vi "rawcdc_protocol.vi"() -> ()   [LabVIEW 2024]
doc: "This example performs writes and reads on a serial port, as directed by the user. You can press the Write and Read buttons, and change the Read Count, while the example is running.\n\nThe parameters set for the serial port must match the parameters of the connected instrument or device. In this example, the Read Count parameter specifies the number of bytes that the serial port reads. If there were more bytes at the port than the specified number, those bytes would not be read. If there were less bytes at the port than the specified number, you would receive a timeout error.\n\nThis example expands upon the flow control options for XON and XOFF, allowing the user to choose those control characters. Also, the user can enable or disable a termination character. Some devices require a termination character in order to identify the end of command strings. Some devices send a termination character to signify the end of data to be read. This example shows how you can end the Read operation once a termination character is detected in the buffer and/or append a termination character at the end of the Write data."
uses:
  <vilib>/Instr/_visa.llb/VISA Configure Serial Port (Instr).vi
panel:
  in  "Correction":dbl(slide) scale=-10.0..10.0
  in  "index (row)":i32
  in  "Cal Array":dbl[][](array[numeric])
  out "Scaled":dbl
  out "Measured":dbl
  out "Waveform Chart":dbl[](graph)
  in  "Command List":string="stop\nencode 0\nslist 0 0\nsrate 6000\nps 2\ndec 1\ndeca 3\nnop\n\n\n"
  in  "Stop":bool
  in  "2108 CDC Virtual COM":refnum<visa-resource-name>="COM11"
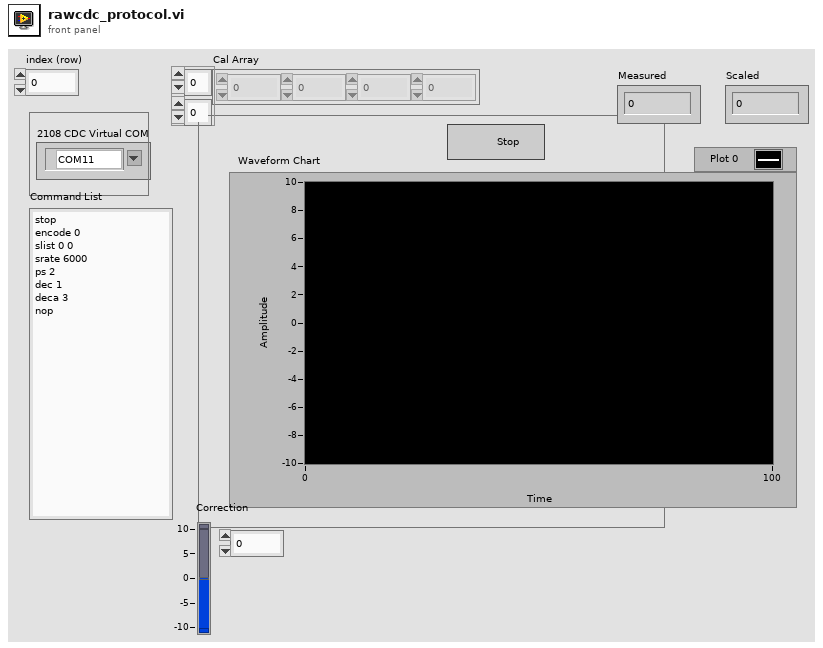
[diagram p1: front panel]
types:
  T1 = enum16{"big-endian, network order", "native, host order", "little-endian"}
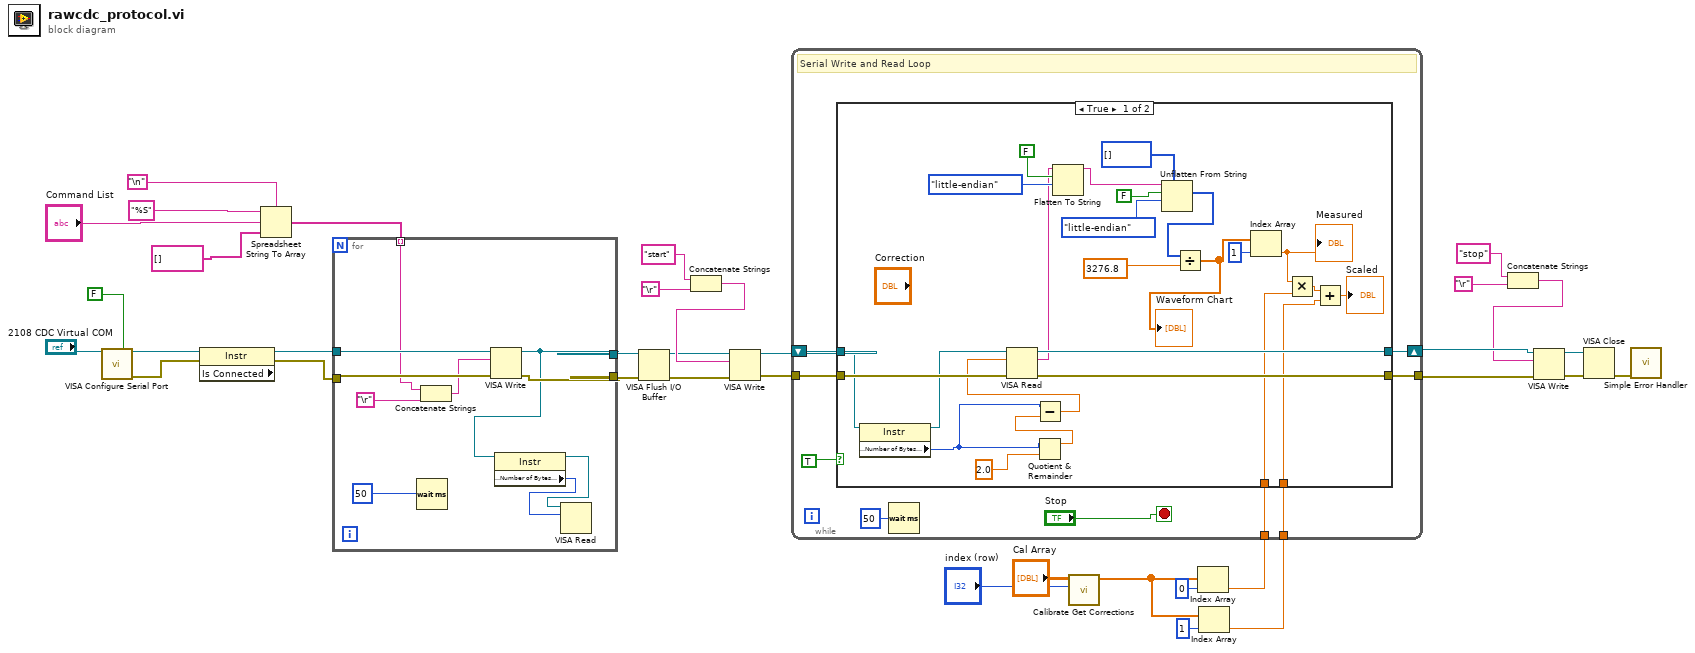
[diagram p0: block diagram]
diagram:
  n1 = call-poly "VISA Configure Serial Port"("VISA resource name"="2108 CDC Virtual COM", "Enable Termination\nChar (T)"=FALSE) -> ("VISA resource name out"=w33:refnum<visa-resource-name>, "error out"=w35:errorcluster)  [unwired: 8 in, 4 out]
  n2 = property class="Instr" props=["Is Connected"](reference=w33, error in=w35) -> (reference out=w9:refnum<visa-resource-name>, error out=w8:errorcluster)  [unwired: 1 out]
  n3 = Spreadsheet String To Array(delimiter (Tab)="\n", format string="%S", spreadsheet string="Command List", array type (2D Dbl)=string[] []) -> (array=w29:string[])
  n4 = for {
    tunnel: w29 -> [w42] mode=indexing
    tunnel: w9 -> [w45]
    tunnel: w8 -> [w44]
    tunnel: [w38] -> w13
    tunnel: [w39] -> w11
    n5 = Wait (ms)(milliseconds to wait=u32 50) -> ()  [unwired: 1 out]
    n6 = Concatenate Strings(w42, "\r") -> (w40:string)
    n7 = VISA Write(VISA resource name=w45, write buffer=w40, error in (no error)=w44) -> (VISA resource name out=w38:refnum<visa-resource-name>, error out=w39:errorcluster)  [unwired: 1 out]
    n8 = property class="Instr"(reference=w38) -> (reference out=w37:refnum<visa-resource-name>, "Serial Settings:Number of Bytes at Serial Port"=w36:u32)  [unwired: 1 in, 1 out]
    n9 = VISA Read(VISA resource name=w37, byte count=w36) -> ()  [unwired: 1 in, 4 out]
  }
  n10 = VISA Flush I/O Buffer(VISA resource name=w13, error in (no error)=w11) -> (VISA resource name out=w12:refnum<visa-resource-name>, error out=w10:errorcluster)  [unwired: 1 in]
  n11 = Concatenate Strings("start", "\r") -> (w17:string)
  n12 = VISA Write(VISA resource name=w12, write buffer=w17, error in (no error)=w10) -> (VISA resource name out=w16:refnum<visa-resource-name>, error out=w15:errorcluster)  [unwired: 1 out]
  n13 = call "Calibrate Get Corrections.vi"("index (row)"="index (row)", "Cal Array"="Cal Array") -> ("Array"=w3:dbl[])  [unwired: 9 in]
  n14 = Index Array(array=w3, index=0) -> (element=w2:dbl)
  n15 = Index Array(array=w3, index=1) -> (element=w1:dbl)
  n16 = while {
    shift-right: [w54] -> w26
    shift-left: w16 -> [w50]
    tunnel: w15 -> [w49]
    tunnel: [w52] -> w23
    tunnel: w2 -> [w47]
    tunnel: w1 -> [w46]
    stop <- "Stop" stop-if-true
    # "Serial Write and Read Loop"
    n17 = case shown="True" TRUE {
      tunnel: [w78 w81] -> w54
      tunnel: w50 -> [w76 w81]
      tunnel: w49 -> [w79 w80]
      tunnel: [w71 w80] -> w52
      tunnel: w47 -> [w56 _]
      tunnel: w46 -> [w55 _]
      frame True {
        n18 = property class="Instr"(reference=w76) -> (reference out=w70:refnum<visa-resource-name>, "Serial Settings:Number of Bytes at Serial Port"=w75:u32)  [unwired: 1 in, 1 out]
        n19 = Quotient & Remainder(x=w75, y=2.0) -> (x-y*floor(x/y)=w73:dbl)  [unwired: 1 out]
        n20 = Subtract(x=w75, y=w73) -> (x-y=w72:dbl)
        n21 = VISA Read(VISA resource name=w70, byte count=w72, error in (no error)=w79) -> (VISA resource name out=w78:refnum<visa-resource-name>, read buffer=w64:string, error out=w71:errorcluster)  [unwired: 1 out]
        n22 = Flatten To String(anything=w64, prepend array or string size? (T)=FALSE, byte order (0:big-endian, network order)=T1."little-endian") -> (data string=w65:string)  [unwired: 1 in, 2 out]
        n23 = Unflatten From String(type=i16[] [], binary string=w65, data includes array or string size? (T)=FALSE, byte order (0:big-endian, network order)=T1."little-endian") -> (value=w63:i16[])  [unwired: 1 in, 2 out]
        n24 = Divide(x=w63, y=3276.8) -> (x/y=w61:dbl[])
        "Waveform Chart" <- w61
        n25 = Index Array(array=w61, index=1) -> (element=w59:dbl)
        "Measured" <- w59
        n26 = Multiply(x=w59, y=w56) -> (x*y=w58:dbl)
        n27 = Add(x=w58, y=w55) -> (x+y=→"Scaled":dbl)
      }
      frame False {
      }
    }
    n28 = Wait (ms)(milliseconds to wait=u32 50) -> ()  [unwired: 1 out]
  }
  n29 = Concatenate Strings("stop", "\r") -> (w20:string)
  n30 = VISA Write(VISA resource name=w26, write buffer=w20, error in (no error)=w23) -> (VISA resource name out=w25:refnum<visa-resource-name>, error out=w24:errorcluster)  [unwired: 1 out]
  n31 = VISA Close(VISA resource name=w25, error in (no error)=w24) -> (error out=w34:errorcluster)
  n32 = call <vilib>:"Simple Error Handler.vi"("error in (no error)"=w34) -> ()  [unwired: 1 in, 8 out]
